vi "getCurrent.vi"(3 "error in (no error)":errorcluster, 4 "Throttle % [0-100]":dbl, 5 "Ammeter Emulator in":refnum<class "Ammeter Emulator.lvclass">) -> (0 "error out":errorcluster, 1 "Current [Amps]":dbl, 2 "Ammeter Emulator out":refnum<class "Ammeter Emulator.lvclass">)   [LabVIEW 2015, in "Ammeter Emulator.lvclass"]
uses:
  Ammeter Emulator.lvclass
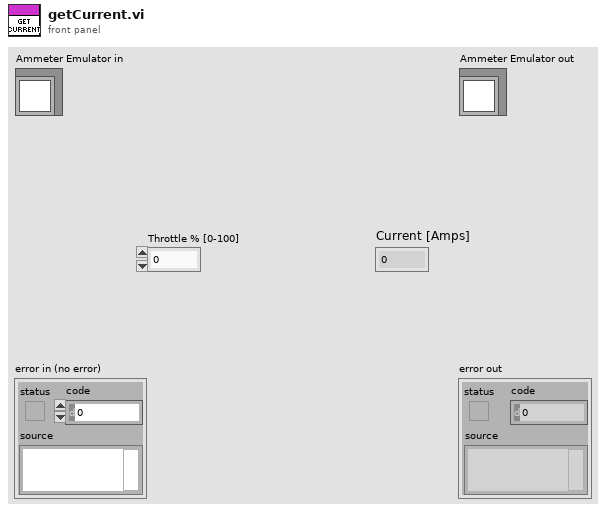
[diagram p1: front panel]
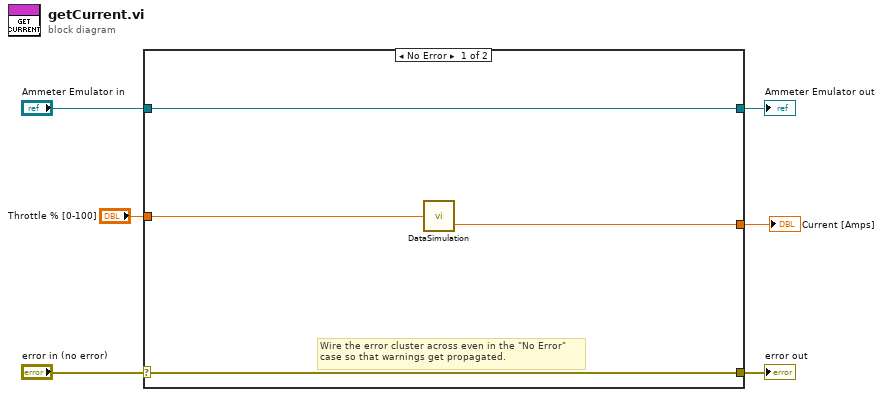
[diagram p0: block diagram]
diagram:
  n1 = case shown="No Error" "error in (no error)" {
    selector: "error in (no error)" -> [w9 w12]
    tunnel: [w9 w12] -> w5
    tunnel: [w10 w11] -> w3
    tunnel: "Ammeter Emulator in" -> [w10 w11]
    tunnel: "Throttle % [0-100]" -> [w8 _]
    tunnel: [w7 _] -> w1
    frame No Error {
      # "Wire the error cluster across even in the \"No Error\"\ncase so that warnings get propagated."
      n2 = call "DataSimulation.vi"("Throttle % [0-100]"=w8) -> ("Amp Draw from Ammeter [Amps]"=w7:dbl)  [unwired: 2 in, 1 out]
    }
    frame Error {
    }
  }
  "error out" <- w5
  "Ammeter Emulator out" <- w3
  "Current [Amps]" <- w1
